vi "SimulatedData.vi"(9 "dt":dbl, 10 "u_delayed":dbl, 11 "T(0)":dbl) -> (2 "T_next":dbl)   [LabVIEW 2025]
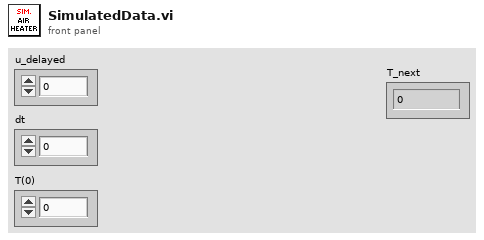
[diagram p1: front panel]
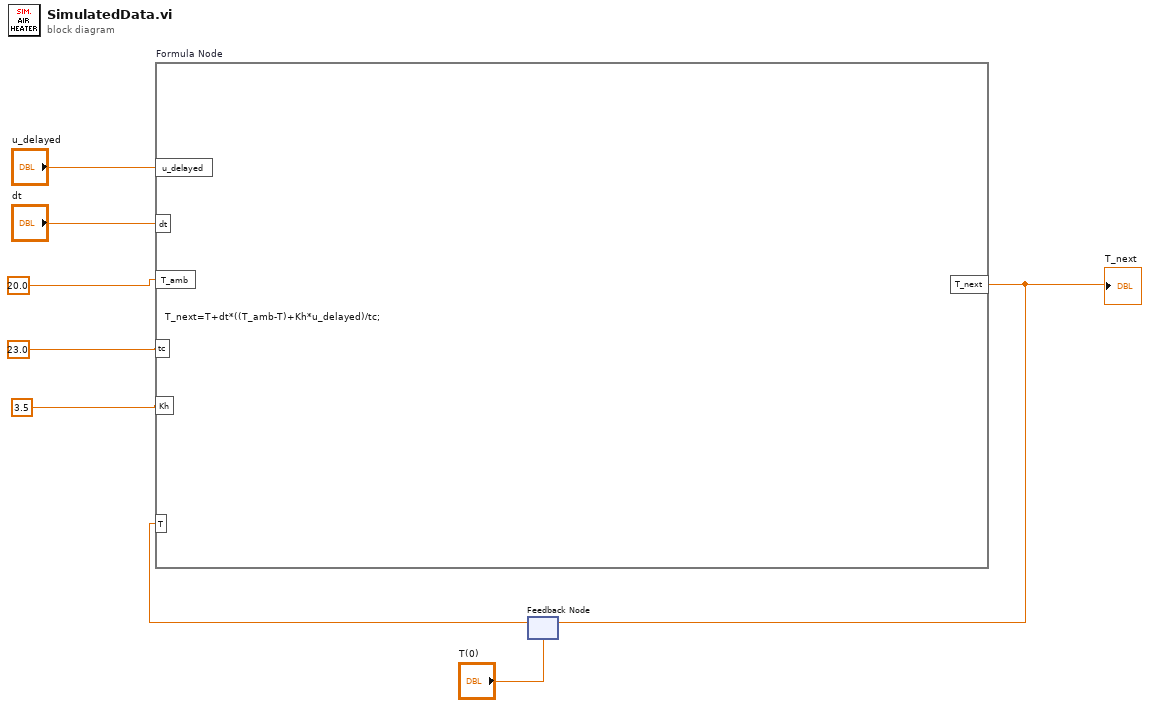
[diagram p0: block diagram]
diagram:
  n1 = feedback #1("T(0)") -> (w2:dbl)
  n2 = formula code="T_next=T+dt*((T_amb-T)+Kh*u_delayed)/tc;"("T"=w2, "u_delayed"="u_delayed", "dt"="dt", "T_amb"=20.0 ("input variable"), "tc"=23.0 ("input variable"), "Kh"=3.5 ("input variable")) -> ("T_next"=w3:dbl)
  "T_next" <- w3
  n3 = feedback-in #1(w3) -> ()
